vi "PH_Sequencer.get Head Information by PU Name.vi"(0 "i ref in":refnum<vi>, 2 "PU Instance Name":string="N/A", 5 "error in (no error)":errorcluster) -> (14 "i ref out":refnum<vi>, 16 "Heads Information as Array":T1[](array[typedef]) {"Information"."State" items=["no info", "off/false/out", "on/true/in", "Failure", "Alarm", "Status 1", "Status 2", "Status 3"]}, 17 "index of power unit":i32, 18 "Head Information":T1={"PowerUnit"=enum."no Info", "GUI Ref"=refnum, "Information"={"State"=2, "Waiting Time [s]"=1800.0, "PU State SM"=enum.".", "PU Timeout SM"=enum."."}, "linked?"=FALSE, "GUI Ref Current Voltage"=refnum} {"Information"."State" items=["no info", "off/false/out", "on/true/in", "Failure", "Alarm", "Status 1", "Status 2", "Status 3"]}, 19 "error out":errorcluster)   [LabVIEW 2014, in "PH_Sequencer.lvlib"]
doc: "This VI gets the index and other head information by the PU Name."
uses:
  PH_Sequencer.lvlib
  PH_Sequencer.Head.ctl
  PH_Basics/PH_PP_Common/PH_PP_Common.PUs.ctl
  PH_Sequencer.PU Information for GUI.ctl
  PH_Basics/PH_StatusHandler/PH_StatusHandler.GUI element.ctl
  PH_Basics/PH_PowerUnit_BaseClass/PH_PowerUnit_BaseClass.SM States.ctl
  PH_Sequencer.PU Information.ctl
  PH_Basics/PH_StatusHandler/PH_StatusHandler.Status.ctl
  PH_Basics/PH_StatusHandler/PH_StatusHandler.lvlib
  PH_Basics/PH_PP_Common/PH_PP_Common.lvlib
  PH_Basics/PH_PowerUnit_BaseClass/PH_PowerUnit_BaseClass.lvlib
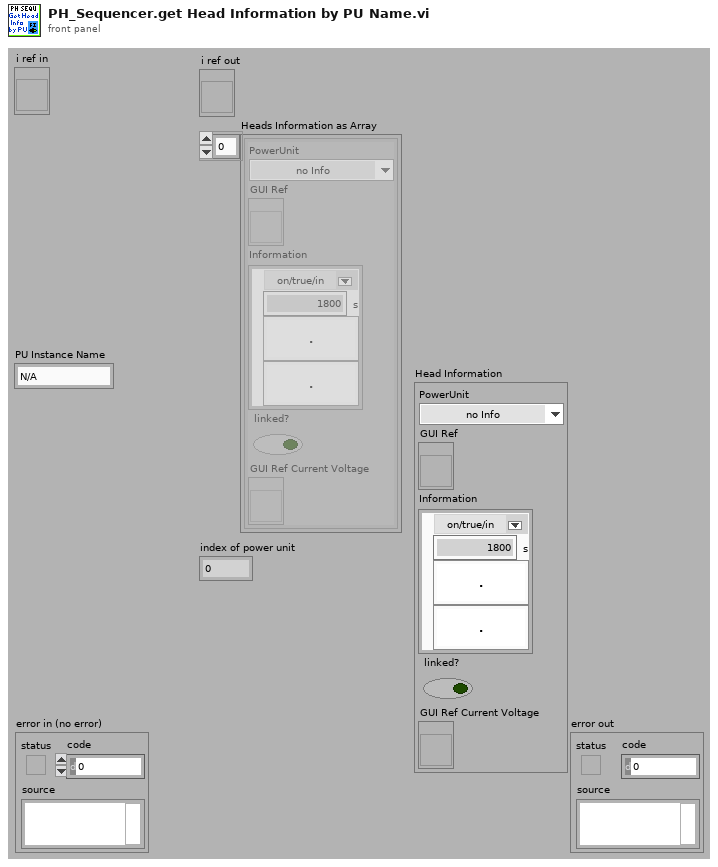
[diagram p1: front panel]
types:
  T1 = typedef "PH_Sequencer.lvlib/PH_Sequencer.Head.ctl" = cluster{"PowerUnit":T2, "GUI Ref":refnum<vi>, "Information":T3, "linked?":bool, "GUI Ref Current Voltage":refnum<vi>}
  T2 = typedef "PH_PP_Common.lvlib/PH_PP_Common.PUs.ctl" = enum16{"no Info", "PA-19mm-1", "PA-19mm-2", "PA-45mm-PILC", "PA-45mm-MAIN", "MA-PU-1", "MA-PU-2", "MA-PU-3", "MA-PU-4", "MA-PU-5", "MA-PU-6", "MA-FR", "MA-PILC", "PA-45mm-DP"}
  T3 = typedef "PH_Sequencer.lvlib/PH_Sequencer.PU Information.ctl" = cluster{"State":T4, "Waiting Time [s]":dbl, "PU State SM":T5, "PU Timeout SM":T5}
  T4 = typedef "PH_StatusHandler.lvlib/PH_StatusHandler.Status.ctl" = i16
  T5 = typedef "PH_PowerUnit_BaseClass.lvlib/PH_PowerUnit_BaseClass.SM States.ctl" = enum16{".", "Stand by", "Switch PU on", "Configure", "Set Default Voltage", "Set STANDBY", "Set READY", "Wait for Shot Cmd", "Open Dump Rods", "Open Ross Relais", "Close Ross Relais", "Switch PSU on", "Switch PSU off", "Charge", "Switch GD Channel on", "Close Dump Rods", "Rods-TO", "RR-TO", "PSU-TO", "Trigger-TO"}
  T6 = typedef "PH_Sequencer.lvlib/PH_Sequencer.i attribute.ctl" = cluster{"GUI Refs":cluster{"Main Off":refnum<vi>, "Fire":refnum<vi>, "Status":refnum<vi>, "Ready":refnum<vi>, "Waiting Time":refnum<vi>, "Timeout":refnum<vi>, "PPMA Ready":refnum<vi>, "Sequencer SM State":refnum<vi>, "PPPA Ready":refnum<vi>, "Calorimeter":refnum<vi>, "Beamline Ready":refnum<vi>, "Clear Beamline":refnum<vi>, "Linkage PPMA Rods":refnum<vi>, "Linkage Current PA":refnum<vi>, "Linkage Current MA":refnum<vi>, "Timing Ready":refnum<vi>, "State Timing":refnum<vi>, "Force Timing":refnum<vi>, "PSDB Shot Comment":refnum<vi>, "State PA Backreflection":refnum<vi>, "Beamline Z6 Ready":refnum<vi>, "Clear Z6 Beamline":refnum<vi>, "Sequence length":refnum<vi>, "Timing Mode":refnum<vi>, "Slow Trigger Settings":refnum<vi>, "Experiment Description":refnum<vi>, "State PSDB":refnum<vi>, "PSDB Ready":refnum<vi>, "Set PSDB Settings":refnum<vi>, "Get PSDB Info":refnum<vi>, "Take Snapshot":refnum<vi>, "Shottype":refnum<vi>, "Experiment":refnum<vi>, "Phase Frontends":refnum<vi>, "PP 45mm PILC in use":refnum<vi>}, "Status Info":cluster{"Machine Status":T4, "WaitingTime":i32, "Timeout":bool}, "Readyness":cluster{"Ready to shot":bool, "PPMA Ready":bool, "PPPA Ready":bool, "BL Ready":bool, "Timing Ready":bool, "BL Z6 Ready":bool, "PSDBReady":bool}, "Instancenames":cluster{"PPMA Rods":string, "PP Current Meas":string, "PH Beamline Chief":string, "PA Backrefl Meas":string, "Z6 Beamline Chief":string}, "Data to read":bool, "Calorimeter":cluster{"Instancename":string, "On":bool, "linked":bool}, "Linkage":cluster{"PPMA Rods":bool, "PP Current Meas":bool, "PHELIX Beamline Chief":bool, "PA Backrefl Meas":bool, "Z6 Beamline Chief":bool}, "Timing":cluster{"Instance":string, "linked":bool, "Status":T4, "Timing Mode":T7, "Slow Trigger Settings":T8, "Info available":cluster{"ext SlowTrigger":bool, "T2":bool, "Mode":bool, "Delay Slow Trigger":bool, "Phase FEs":bool}, "FE Phase":T9}, "Service ID R2S":i32, "PSDB":cluster{"Controller Instance":string, "Controller Status":T4, "Controller linked":bool, "Settings acknowledged":bool, "Current Experiment ID":i16, "Current Shot Type":i16, "Current Comment":string, "Remember Settings":bool, "Write 2 early":bool}, "PSDB Data":cluster{"Main Off?":bool, "Sequence Length":dbl, "Sequence startet":timestamp}, "6P 4Q Positions":cluster{"Instancename":string, "linked":bool, "Position":T10}[], "PUs":T1[]}
  T7 = typedef "PH_Timing.lvlib/PH_Timing.Timing Mode.ctl" = cluster{"T2":i16, "Modeselector":enum32{"10 Hz", "0.5 Hz", "Shot"}}
  T8 = typedef "PH_Timing.lvlib/PH_Timing.Slow Trigger Settings.ctl" = cluster{"Delay":dbl, "externally triggered?":bool}
  T9 = typedef "PH_Timing.lvlib/PH_Timing.Phase FEs.ctl" = cluster{"Phase":dbl}
  T10 = typedef "PH_4_Pos_Selector.lvlib/PH_4_Pos_Selector.Position Selector.ctl" = u16
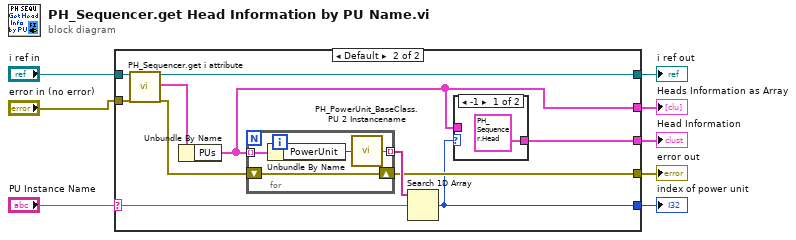
[diagram p0: block diagram]
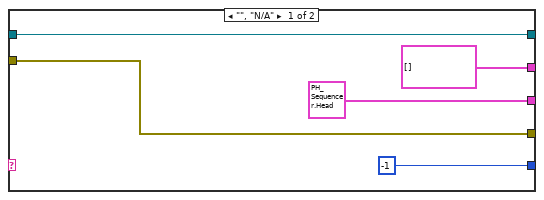
[diagram p2: hidden frame]
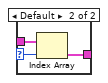
[diagram p3: hidden frame]
diagram:
  n1 = case shown="Default" "PU Instance Name" {
    selector: "PU Instance Name" -> [_ w17]
    tunnel: "error in (no error)" -> [w12 w23]
    tunnel: [w13 w22] -> w7
    tunnel: "i ref in" -> [w13 w21]
    tunnel: [T1[] [] ("Heads") w14] -> w5
    tunnel: [-1 ("index of element") w15] -> w4
    tunnel: [T1 {"PowerUnit"=enum."no Info", "GUI Ref"=refnum, "Information"={"State"=0, "Waiting Time [s]"=0.0, "PU State SM"=enum.".", "PU Timeout SM"=enum."."}, "linked?"=FALSE, "GUI Ref Current Voltage"=refnum} ("PA 19mm - 1") w16] -> w3
    tunnel: [w12 w18] -> w2
    frame "", "N/A" {
    }
    frame Default {
      n2 = call "PH_Sequencer.get i attribute.vi"("i ref in"=w21, "error in (no error)"=w23) -> ("i ref out"=w22:refnum<vi>, "i attribute"=w24:T6, "error out"=w19:errorcluster)  [unwired: 15 in]
      n3 = Unbundle By Name(w24) -> ("PUs"=w14:T1[])
      n4 = for {
        tunnel: w14 -> [w32] mode=indexing
        tunnel: [w29] -> w20 mode=indexing
        shift-right: [w31] -> w18
        shift-left: w19 -> [w31]
        n5 = Unbundle By Name(w32) -> ("PowerUnit"=w30:T2)
        n6 = call "PH_PowerUnit_BaseClass.PU 2 Instancename.vi"("PU"=w30) -> ("Instance Name"=w29:string)
      }
      n7 = Search 1D Array(1D array=w20, element=w17) -> (index of element=w15:i32)  [unwired: 1 in]
      n8 = case shown="-1" w15 {
        selector: w15 -> [_ w26]
        tunnel: w14 -> [_ w28]
        tunnel: [T1 {"PowerUnit"=enum."no Info", "GUI Ref"=refnum, "Information"={"State"=0, "Waiting Time [s]"=0.0, "PU State SM"=enum.".", "PU Timeout SM"=enum."."}, "linked?"=FALSE, "GUI Ref Current Voltage"=refnum} ("PA 19mm - 1") w27] -> w16
        frame -1 {
        }
        frame Default {
          n9 = Index Array(array=w28, index=w26) -> (element=w27:T1)
        }
      }
    }
  }
  "error out" <- w2
  "i ref out" <- w7
  "index of power unit" <- w4
  "Heads Information as Array" <- w5
  "Head Information" <- w3
